vi "Set All Names and Values.vi"(6 "Cluster Name":string, 8 "error in":errorcluster, 9 "values":variant[](array[variant]), 10 "Element Names":string[](array[string]), 11 "Cluster in":variant) -> (0 "error out":errorcluster, 3 "Cluster out":variant)   [LabVIEW 2020, in "Variant Data Manipulation.lvlib"]
doc: "Returns an array of all of the keys and an array of their corresponding values. Elements are correlated by index, so the key at a given index corresponds to the value at the same index."
uses:
  Variant Data Manipulation.lvlib
  <vilib>/Utility/Data Type/NI_Data Type.lvlib
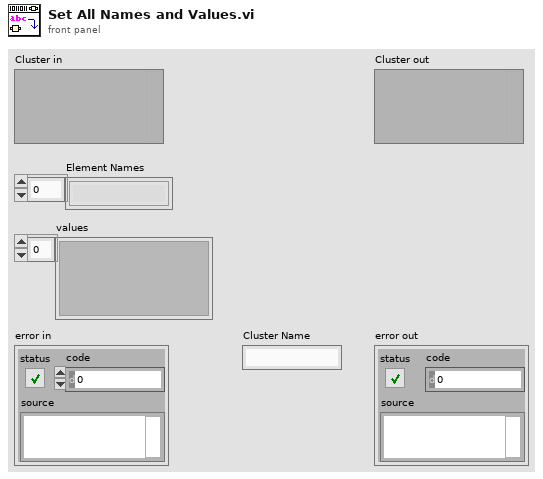
[diagram p1: front panel]
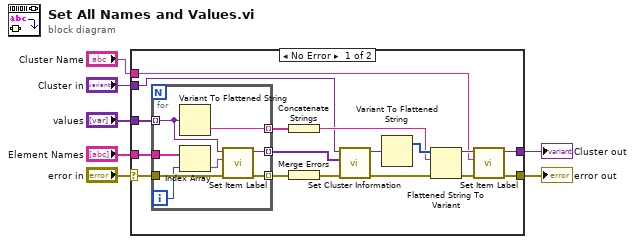
[diagram p0: block diagram]
diagram:
  n1 = case shown="No Error" "error in" {
    selector: "error in" -> [w13 w33]
    tunnel: "Cluster in" -> [w10 w34]
    tunnel: "values" -> [w18 _]
    tunnel: [w15 w34] -> w5
    tunnel: [w14 w33] -> w3
    tunnel: "Element Names" -> [w19 _]
    tunnel: "Cluster Name" -> [w8 _]
    frame No Error {
      n2 = for {
        tunnel: w18 -> [w29] mode=indexing
        tunnel: [w32] -> w24 mode=indexing
        tunnel: w19 -> [w31]
        tunnel: [w30] -> w17 mode=indexing
        tunnel: w13 -> [w28]
        tunnel: [w27] -> w12 mode=indexing
        i -> [w25]
        n3 = Variant To Flattened String(Variant=w29) -> (data string=w32:string)  [unwired: 1 out]
        n4 = Index Array(array=w31, index=w25) -> (element=w26:string)
        n5 = call "Set Item Label.vi"("error in (no error)"=w28, "Name"=w26, "Variant in"=w29) -> ("error out"=w27:errorcluster, "Variant out"=w30:variant)  [unwired: 7 in]
      }
      n6 = Concatenate Strings(w24) -> (w21:string)
      n7 = Merge Errors(w12) -> (w11:errorcluster)
      n8 = call <vilib>:"Set Cluster Information.vi"("error in (no error)"=w11, "Cluster Elements"=w17, "Variant in"=w10) -> ("error out"=w20:errorcluster, "Variant out"=w23:variant)  [unwired: 7 in]
      n9 = Variant To Flattened String(Variant=w23) -> (1:w22:i16[])  [unwired: 1 out]
      n10 = Flattened String To Variant(4:w20, 6:w21, 7:w22) -> (0:w9:errorcluster, 3:w16:variant)
      n11 = call "Set Item Label.vi"("error in (no error)"=w9, "Name"=w8, "Variant in"=w16) -> ("error out"=w14:errorcluster, "Variant out"=w15:variant)  [unwired: 7 in]
    }
    frame Error {
    }
  }
  "error out" <- w3
  "Cluster out" <- w5
